vi "sub UI set bp.vi"(8 "error in (no error)":errorcluster, 10 "<bp> data":T1, 11 "IDE simple in":refnum<class "LF2R IDE.lvclass">) -> (0 "error out":errorcluster, 3 "IDE simple out":refnum<class "LF2R IDE.lvclass">)   [LabVIEW 2018, in "LF2R IDE.lvlib" / "LF2R IDE.lvclass"]
uses:
  LF2R IDE.lvclass
  Frame Analizer/frame bp data.ctl
  LF2R IDE.lvclass/LF2R IDE.ctl
  Frame Analizer/Data Parser.lvclass
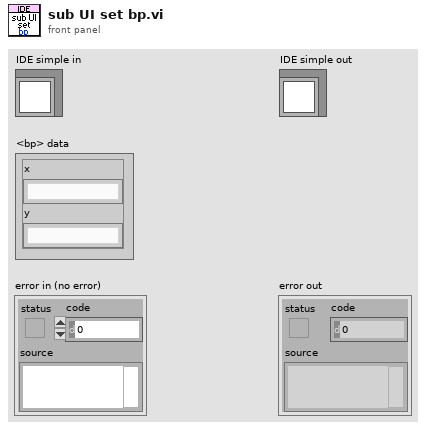
[diagram p1: front panel]
types:
  T1 = typedef "Data Parser.lvclass/frame bp data.ctl" = cluster{"x":string, "y":string}
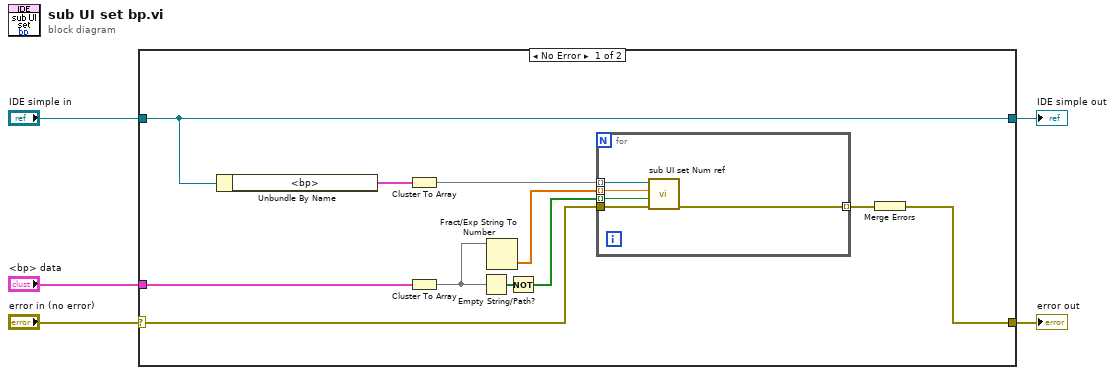
[diagram p0: block diagram]
diagram:
  n1 = case shown="No Error" "error in (no error)" {
    selector: "error in (no error)" -> [w14 w23]
    tunnel: [w9 w23] -> w4
    tunnel: [w11 w22] -> w2
    tunnel: "IDE simple in" -> [w11 w22]
    tunnel: "<bp> data" -> [w7 _]
    frame No Error {
      n2 = Unbundle By Name(w11) -> ("<bp>"=w16:cluster{"x":refnum<vi>, "y":refnum<vi>})
      n3 = Cluster To Array(cluster=w16) -> (array=w8:refnum<vi>[])
      n4 = Cluster To Array(cluster=w7) -> (array=w6:string[])
      n5 = Empty String/Path?(string/path=w6) -> (empty?=w15:bool[])
      n6 = Fract/Exp String To Number(string=w6) -> (number=w12:dbl[])  [unwired: 3 in, 1 out]
      n7 = Not(x=w15) -> (.not. x?=w13:bool[])
      n8 = for {
        tunnel: w14 -> [w21]
        tunnel: w8 -> [w18] mode=indexing
        tunnel: w13 -> [w17] mode=indexing
        tunnel: w12 -> [w20] mode=indexing
        tunnel: [w19] -> w10 mode=indexing
        n9 = call "sub UI set Num ref.vi"("error in"=w21, "valid"=w17, "Value"=w20, "num ref"=w18) -> ("error out"=w19:errorcluster)  [unwired: 7 in]
      }
      n10 = Merge Errors(w10) -> (w9:errorcluster)
    }
    frame Error {
    }
  }
  "error out" <- w4
  "IDE simple out" <- w2
